vi "Check Execution Unit Channel Count.vi"(7 "Channel Counts":T1={"Incoming"=34, "Outgoing"=34, "ReadWrite"=34}, 8 "error in":errorcluster, 10 "Execution Unit Information":T2 {"ReadWrite Channels" format="%.0x"; "Outgoing Channels" format="%.0x"; "Incoming Channels" format="%.0x"}, 11 "TestCase in":refnum<class "Create Execution Unit.lvclass">) -> (0 "error out":errorcluster, 2 "Execution Unit":refnum<class "Execution Unit.lvclass">, 3 "TestCase out":refnum<class "Create Execution Unit.lvclass">)   [LabVIEW 2020, in "Create Execution Unit.lvclass"]
uses:
  Create Execution Unit.lvclass
  Engine/Interfaces/Controls/Execution Unit Information.ctl
  Engine/Interfaces/Execution Unit/Execution Unit.lvclass
  <vilib>/NI VeriStand/Custom Device API/Custom Device Item Ref.ctl
  <vilib>/NI VeriStand/Custom Device API/Custom Device API.lvlib
  Engine/Interfaces/Interfaces.lvlib
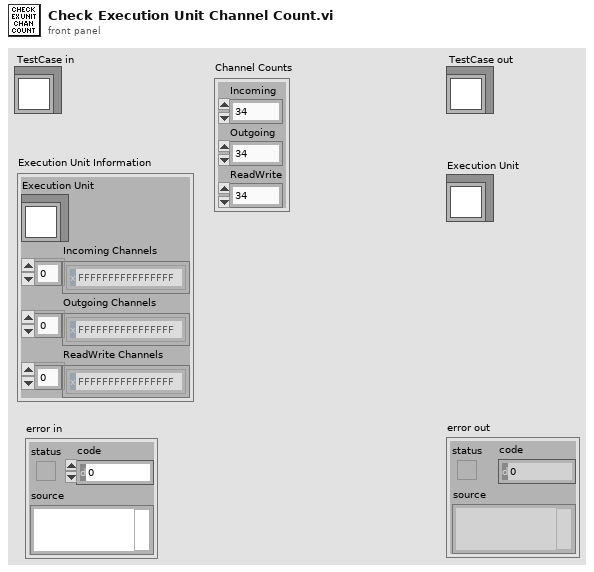
[diagram p1: front panel]
types:
  T1 = cluster{"Incoming":i32, "Outgoing":i32, "ReadWrite":i32}
  T2 = typedef "AIM MIL-STD-1553 Engine.lvlib/Interfaces.lvlib/Execution Unit Information.ctl" = cluster{"Execution Unit":refnum<class "Execution Unit.lvclass">, "Incoming Channels":T3[], "Outgoing Channels":T3[], "ReadWrite Channels":T3[]}
  T3 = typedef "Custom Device API.lvlib/Custom Device Item Ref.ctl" = u64
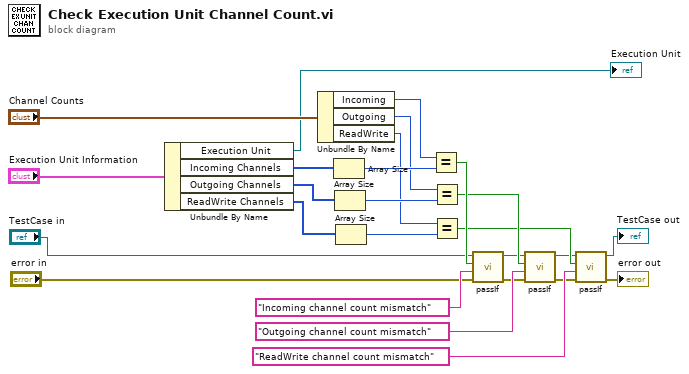
[diagram p0: block diagram]
diagram:
  n1 = Unbundle By Name("Execution Unit Information") -> ("Execution Unit"=→"Execution Unit":refnum<class "Execution Unit.lvclass">, "Incoming Channels"=w22:T3[], "Outgoing Channels"=w23:T3[], "ReadWrite Channels"=w24:T3[])
  n2 = Unbundle By Name("Channel Counts") -> ("Incoming"=w21:i32, "Outgoing"=w19:i32, "ReadWrite"=w17:i32)
  n3 = Array Size(array=w22) -> (size(s)=w20:i32)
  n4 = Array Size(array=w23) -> (size(s)=w18:i32)
  n5 = Array Size(array=w24) -> (size(s)=w16:i32)
  n6 = Equal?(x=w21, y=w20) -> (x = y?=w15:bool)
  n7 = Equal?(x=w19, y=w18) -> (x = y?=w12:bool)
  n8 = Equal?(x=w17, y=w16) -> (x = y?=w10:bool)
  n9 = call-dynamic "passIf.vi"("error in (no error)"="error in", "message (\"\")"="Incoming channel count mismatch" ("message (\"\")"), "pass"=w15, "TestCase in"="TestCase in") -> ("error out"=w8:errorcluster, "TestCase out"=w2:refnum<class "Create Execution Unit.lvclass">)  [unwired: 6 in]
  n10 = call-dynamic "passIf.vi"("error in (no error)"=w8, "message (\"\")"="Outgoing channel count mismatch" ("message (\"\")"), "pass"=w12, "TestCase in"=w2) -> ("error out"=w9:errorcluster, "TestCase out"=w3:refnum<class "Create Execution Unit.lvclass">)  [unwired: 6 in]
  n11 = call-dynamic "passIf.vi"("error in (no error)"=w9, "message (\"\")"="ReadWrite channel count mismatch" ("message (\"\")"), "pass"=w10, "TestCase in"=w3) -> ("error out"=→"error out":errorcluster, "TestCase out"=→"TestCase out":refnum<class "Create Execution Unit.lvclass">)  [unwired: 6 in]
